vi "HW Configuration.vi"(8 "error in (no error)":errorcluster, 11 "Configuration in":refnum<class "Configuration.lvclass">) -> (0 "error out":errorcluster, 3 "Configuration out":refnum<class "Configuration.lvclass">)   [LabVIEW 2017, in "Hardware.lvlib" / "DAQ Configuration.lvclass"]
uses:
  Hardware/DAQ/config/DAQ Configuration.lvclass
  <userlib>/Configuration Dialog Actor/Configuration.lvclass
  C:/Program Files (x86)/National Instruments/LabVIEW 2017/user.lib/Configuration Dialog Actor/Configuration.lvclass
  Hardware/DAQ/config/DAQ Configuration.lvclass/DAQ Configuration.ctl
panel:
  in  "Type":string(combo)
  in  "Range":cluster{"Ranve (min)":dbl, "Range Max":dbl}
  in  "Sample Rate":dbl
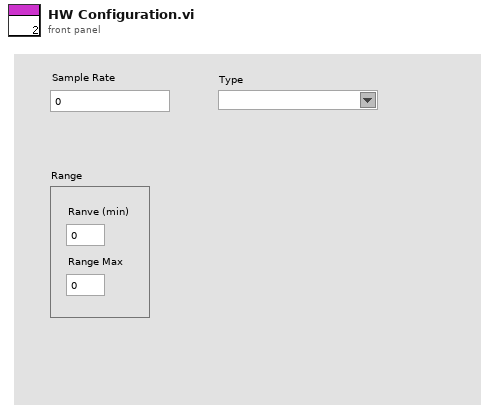
[diagram p1: front panel]
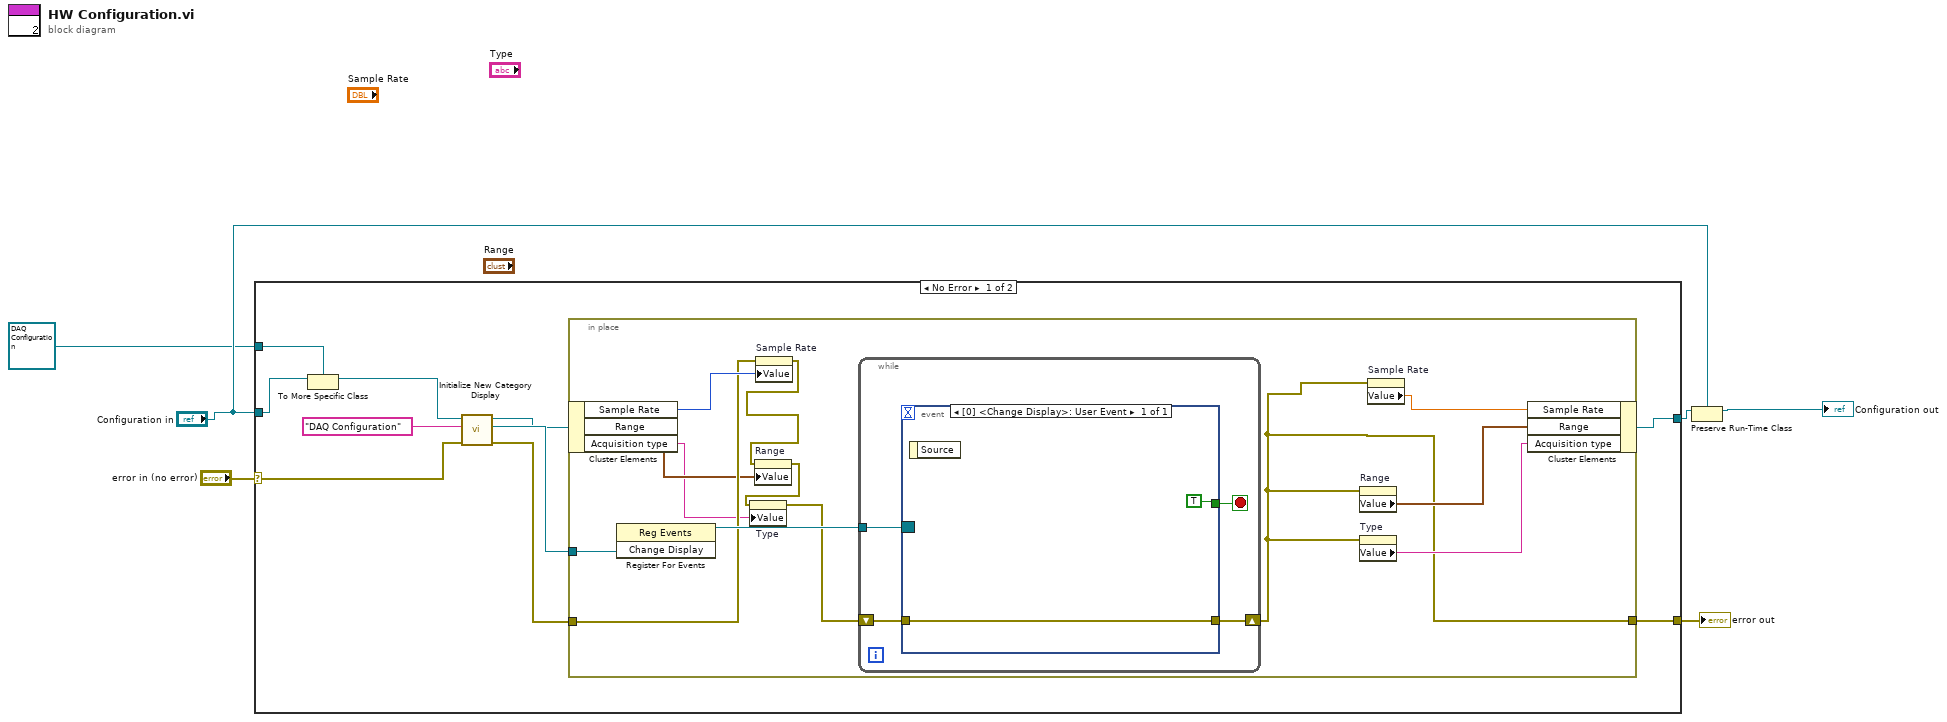
[diagram p0: block diagram]
diagram:
  n1 = case shown="No Error" "error in (no error)" {
    selector: "error in (no error)" -> [w12 w37]
    tunnel: [w11 w36] -> w3
    tunnel: [w14 w37] -> w6
    tunnel: "Configuration in" -> [w10 w36]
    tunnel: refnum<class "DAQ Configuration.lvclass"> refnum ("Hardware.lvlib:DAQ Configuration.lvclass") -> [w8 _]
    frame No Error {
      n2 = To More Specific Class(target class=w8, reference=w10) -> (specific class reference=w9:refnum<class "DAQ Configuration.lvclass">)  [unwired: 1 in, 1 out]
      n3 = call <userlib>:"Initialize New Category Display.vi"("error in (no error)"=w12, "Name to Display"="DAQ Configuration", "Configuration in"=w9) -> ("error out"=w15:errorcluster, "Change Display"=w16:refnum<user-event>, "Configuration Out"=w7:refnum<class "DAQ Configuration.lvclass">)  [unwired: 6 in]
      n4 = in-place {
        in-place-border: w16 -> [w29]
        in-place-border: w15 -> [w26]
        in-place-border: [w17] -> w14
        n5 = in-place-cluster #1(w7) -> ("Sample Rate"=w27:i32, "Range"=w24:cluster{"Ranve (min)":dbl, "Range Max":dbl}, "Acquisition type"=w22:string)
        n6 = register-events(w29) -> (reference out=w28:refnum<event-registration>)  [unwired: 2 in, 1 out]
        n7 = property on="Sample Rate" class="DigNum (strict)"(error in=w26, "Value"=w27) -> (error out=w18:errorcluster)  [unwired: 1 in, 1 out]
        n8 = property on="Range" class="Clust (strict)"(error in=w18, "Value"=w24) -> (error out=w21:errorcluster)  [unwired: 1 in, 1 out]
        n9 = property on="Type" class="CmbBox"(error in=w21, "Value"=w22) -> (error out=w20:errorcluster)  [unwired: 1 in, 1 out]
        n10 = while {
          tunnel: w28 -> [w32]
          shift-right: [w31] -> w17
          shift-left: w20 -> [w30]
          stop <- w33 stop-if-true
          n11 = event shown="[0] <Change Display>: User Event" {
            selector: w32 -> [_]
            dyn-events: _ -> [_]
            timeout: _ -> [_]
            tunnel: [TRUE] -> w33
            tunnel: [w34] -> w31
            tunnel: w30 -> [w34]
            event User Event {
              n12 = event-data() -> ()  [unwired: 1 in, 1 out]
            }
          }
        }
        n13 = property on="Range" class="Clust (strict)"(error in=w17) -> ("Value"=w23:cluster{"Ranve (min)":dbl, "Range Max":dbl})  [unwired: 1 in, 2 out]
        n14 = property on="Type" class="CmbBox"(error in=w17) -> ("Value"=w19:string)  [unwired: 1 in, 2 out]
        n15 = property on="Sample Rate" class="DigNum (strict)"(error in=w17) -> ("Value"=w25:dbl)  [unwired: 1 in, 2 out]
        n16 = in-place-cluster #1("Sample Rate"=w25, "Range"=w23, "Acquisition type"=w19) -> (w11:refnum<class "DAQ Configuration.lvclass">)
      }
    }
    frame Error {
    }
  }
  "error out" <- w6
  n17 = Preserve Run-Time Class(object in=w3, 2:"Configuration in") -> (object out=→"Configuration out":refnum<class "Configuration.lvclass">)  [unwired: 1 in, 1 out]
